vi "Test 7.vi"() -> ()   [LabVIEW 2019]
panel:
  out "最低有效位进位":bool
  out "值 2":i32
  in  "值":i32
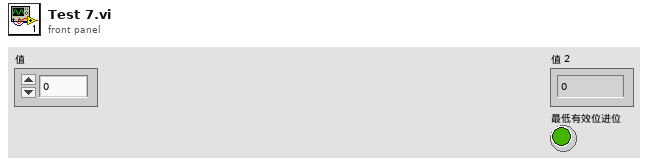
[diagram p1: front panel]
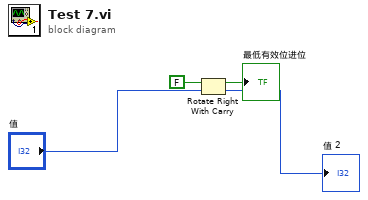
[diagram p0: block diagram]
diagram:
  n1 = Rotate Right With Carry(2:"值", 3:FALSE ("进位")) -> (0:→"值 2":i32, 1:→"最低有效位进位":bool)
